vi "Plot_Current_Measurement_Data.vi"() -> ()   [LabVIEW 2022 SP3]
uses:
  Anemometry Sub Vis/Globals/Meas_global.vi
panel:
  in  "Listbox":i32[](listbox)
  in  "Index 2 scale":dbl=1.0
  out "XY Graph":cluster{"Time (s)":dbl[], "Eng Values":dbl[]}[](graph)
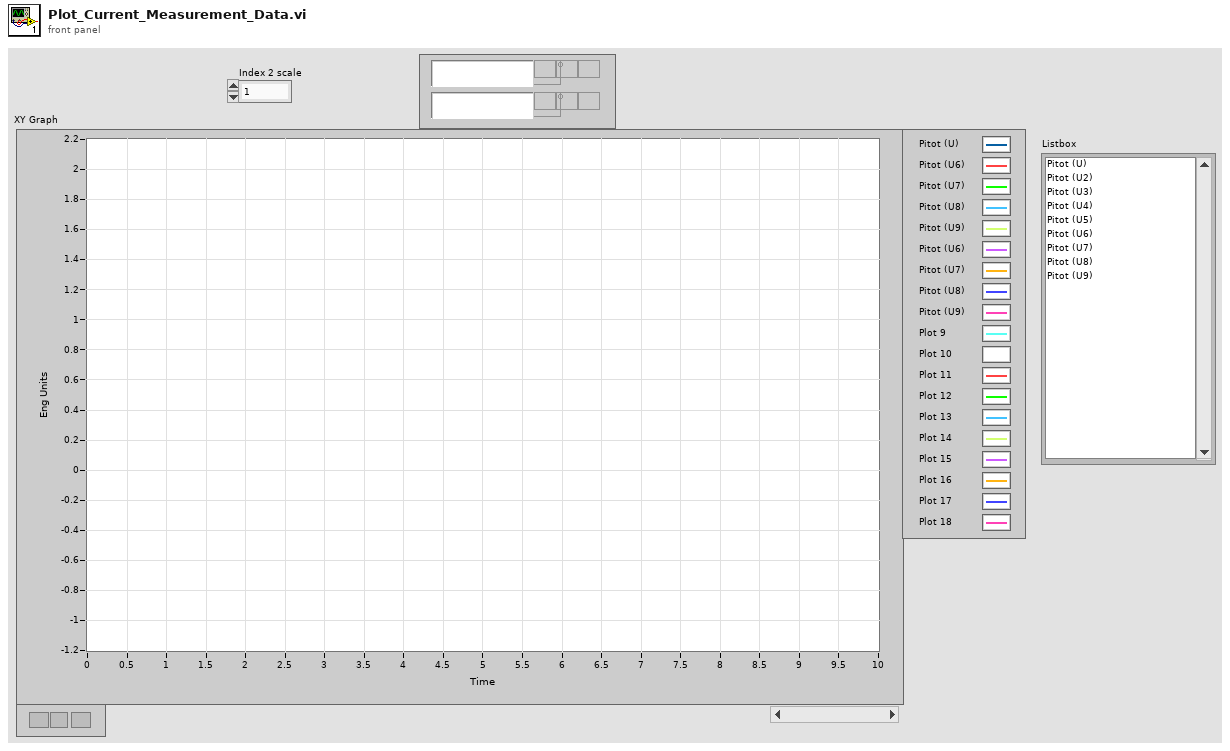
[diagram p1: front panel]
types:
  T1 = typedef "Analysis_info_cluster.ctl" = cluster{"Colour":u32, "Inst type":T2, "Inst name":string, "Symbol":string, "Code name":string, "Extra Info":string, "Inst Array":T3, "Extra Titles":string[], "Extra Values":string[], "U":dbl, "u^2":dbl, "u^3":dbl, "u^4":dbl, "Skew_u":dbl, "Kurt_u":dbl, "Sd Error in Mean":dbl, "% u'/U":dbl, "X":dbl, "Y":dbl, "Z":dbl, "Timescale integral Estimate":dbl, "Sd Error in Variance":dbl, "Calib File":path, "Calib Constants":dbl[], "Output Position":bool, "Stats":enum16{"None", "Basic", "Full"}, "Av Sampling Rate":dbl, "Av No of Samples":dbl, "Total Meas Time (s)":dbl, "ADAM Ch Name":string, "Max value":dbl, "Min value":dbl, "Req Sample Rate Hz":dbl, "Sync Delay Time (s)":dbl, "Ch No":i16, "Device":string, "Use Latest Calib":bool, "Port":string, "Metadata Ch Names":string[], "Metadata Ch Values":string[], "Label":string}
  T2 = typedef "Inst_type.ctl" = enum16{"Raw voltage", "Raw with zero offsetting", "Propeller anemometer", "Pressure Transducer", "Pitot-static tube", "Hot wire", "Cross wire 1", "Cross wire 2", "Generic Linear", "Generic Polynomial", "Generic BackPoly", "Fast FID", "Thermocouple", "Cold wire", "Pulsed Wire", "LDA Vel", "LDA Tran time", "LDA Arr time", "Microphone"}
  T3 = typedef "Instrument_Array.ctl" = enum16{"PWA", "LDA", "Analogue"}
  T4 = typedef "Time_Trace_Cluster.ctl" = cluster{"Weighting":dbl[], "Voltage":dbl[], "Eng Values":dbl[]}
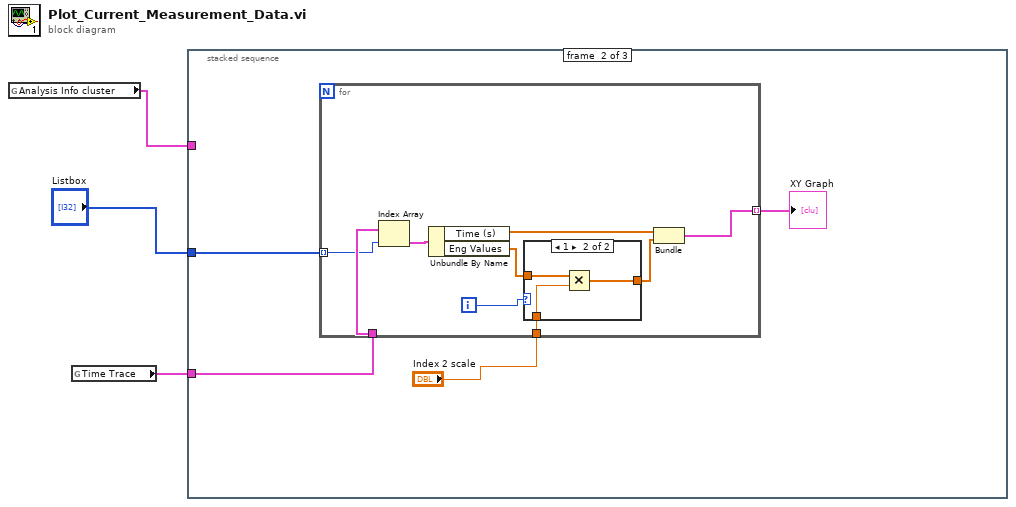
[diagram p0: block diagram]
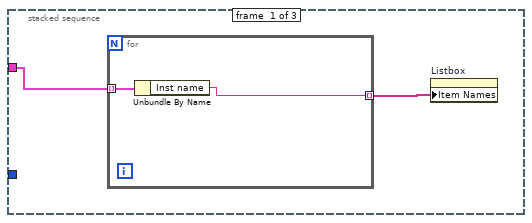
[diagram p2: hidden frame]
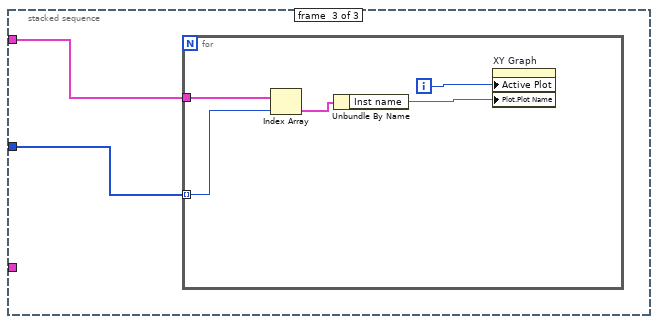
[diagram p4: hidden frame]
diagram:
  n1 = global read "Meas_global.vi" "Analysis Info cluster"() -> (w3:T1[])
  n2 = global read "Meas_global.vi" "Time Trace"() -> (w2:T4[])
  n3 = stacked-sequence {
    tunnel: w3 -> [w5 _ w26]
    tunnel: w2 -> [_ w11 _]
    tunnel: "Listbox" -> [_ w8 w25]
    frame #0 {
      n4 = for {
        tunnel: w5 -> [w7] mode=indexing
        tunnel: [w6] -> w4 mode=indexing
        n5 = Unbundle By Name(w7) -> ("Inst name"=w6:string)
      }
      n6 = property on="Listbox" class="LstBox (strict)"("Item Names"=w4) -> ()  [unwired: 2 in, 2 out]
    }
    frame #1 {
      n7 = for {
        tunnel: w11 -> [w18]
        tunnel: [w17] -> w10 mode=indexing
        tunnel: "Index 2 scale" -> [w15]
        tunnel: w8 -> [w13] mode=indexing
        i -> [w12]
        n8 = Index Array(array=w18, index=w13) -> (element=w19:T4)
        n9 = Unbundle By Name(w19) -> ("Time (s)"=w20:dbl[], "Eng Values"=w16:dbl[])
        n10 = case shown="1" w12 {
          tunnel: w16 -> [w21 w24]
          tunnel: w15 -> [_ w23]
          tunnel: [w21 w22] -> w14
          frame 0, Default {
          }
          frame 1 {
            n11 = Multiply(x=w24, y=w23) -> (x*y=w22:dbl[])
          }
        }
        n12 = Bundle("Time (s)"=w20, "Eng Values"=w14) -> (w17:cluster{"Time (s)":dbl[], "Eng Values":dbl[]})  [unwired: 1 in]
      }
      "XY Graph" <- w10
    }
    frame #2 {
      n13 = for {
        tunnel: w26 -> [w30]
        tunnel: w25 -> [w28] mode=indexing
        i -> [w27]
        n14 = Index Array(array=w30, index=w28) -> (element=w29:T1)
        n15 = Unbundle By Name(w29) -> ("Inst name"=w31:string)
        n16 = property on="XY Graph" class="XYGraph (strict)"("Active Plot"=w27, "Plot.Plot Name"=w31) -> ()  [unwired: 2 in, 2 out]
      }
    }
  }
